vi "top_read_input.vi"(8 "error in (no error)":errorcluster, 10 "Dynamic data":T1, 11 "Input parameters":T2={"Measurement type"=enum."Debug", "Sensor type"=enum."HPK_8in_271ch", "Identifier"="test.txt", "Open after execution?"=FALSE, "Plot after execution?"=FALSE, "Display channel"=0, "Voltage Delay (s)"=0.5, "Switch Delay (s)"=0.01, "VISA resource name source"="", "VISA resource name DMM"="", "VISA resource name LCR"="", "Compliance  Level (A)"=10.0, "Voltage Limit (V)"=1000.0, "Data storage location"="", "Scan voltages"="", "Use source as DMM?"=FALSE, "LCR signal frequenzy (Hz)"=10.0, "DMM device"=enum."Keithley2001", "Sampling number"=1, "Use env. sensors on"=enum."Sensirion sht1x/7x", "Switchboard Handle"=0, "Use Switchboard"=FALSE, "LCR signal voltage (V)"=10000.0, "Repeat"=1, "Scan voltages IV"="", "Scan voltages CV"="", "Hex pad numbers?"=FALSE, "Set measurement type"=enum."Debug", "Custom pad scan"="", "IV voltage Delay (s)"=0.5, "CV voltage Delay (s)"=0.5, "Needle measurement?"=FALSE, "Comments"="test.txt", "LCR signal frequenzy (kHz)"=10.0, "Compliance  Level (uA)"=10.0, "Open Correction Array"=array2304x3[6912 elements], "Current set voltage"=0.0, "Last set voltage"=0.0, "Current channel"=0, "Last OpenCorrection index"=-1, "Total curr/vltg every x steps"=10, "Current channel iteration"=0, "No CV corrections"=FALSE, "Mapfile"="", "Corrfile"="", "IV voltage file"=path "", "CV voltage file"=path "", "IV Switch Delay (s)"=0.01, "CV Switch Delay (s)"=0.01, "Invert polarity"=FALSE, "Set debug dirs"=FALSE, "Is n on p"=FALSE, "Source interlock?"=TRUE, "Voltage file used?"=FALSE, "Pad mask"="", "Mask pad above (uA)"=1.0, "LCR device"=enum."LCR_E4980", "Source device"=enum."Source_2410", "HexPlot binary path"="", "PadReductionFactor"=1.0, "Temperature degC"="", "Fluence [neq]"="", "Annealing [min]"=""} {"CV Switch Delay (s)" format="%#_13g"; "IV Switch Delay (s)" format="%#_13g"; "Last set voltage" format="%#_13g"; "Current set voltage" format="%#_13g"; "CV voltage Delay (s)" format="%#_13g"; "IV voltage Delay (s)" format="%#_13g"; "Voltage Limit (V)" format="%#_13g"; "Voltage Delay (s)" format="%#_13g"; "Switch Delay (s)" format="%#_13g"}) -> (0 "error out":errorcluster, 2 "Dynamic data":T1, 3 "Input parameters":T2={"Measurement type"=enum."Debug", "Sensor type"=enum."HPK_8in_271ch", "Identifier"="test.txt", "Open after execution?"=FALSE, "Plot after execution?"=FALSE, "Display channel"=0, "Voltage Delay (s)"=0.5, "Switch Delay (s)"=0.01, "VISA resource name source"="", "VISA resource name DMM"="", "VISA resource name LCR"="", "Compliance  Level (A)"=10.0, "Voltage Limit (V)"=1000.0, "Data storage location"="", "Scan voltages"="", "Use source as DMM?"=FALSE, "LCR signal frequenzy (Hz)"=10.0, "DMM device"=enum."Keithley2001", "Sampling number"=1, "Use env. sensors on"=enum."Sensirion sht1x/7x", "Switchboard Handle"=0, "Use Switchboard"=FALSE, "LCR signal voltage (V)"=10000.0, "Repeat"=1, "Scan voltages IV"="", "Scan voltages CV"="", "Hex pad numbers?"=FALSE, "Set measurement type"=enum."Debug", "Custom pad scan"="", "IV voltage Delay (s)"=0.5, "CV voltage Delay (s)"=0.5, "Needle measurement?"=FALSE, "Comments"="test.txt", "LCR signal frequenzy (kHz)"=10.0, "Compliance  Level (uA)"=10.0, "Open Correction Array"=array2304x3[6912 elements], "Current set voltage"=0.0, "Last set voltage"=0.0, "Current channel"=0, "Last OpenCorrection index"=-1, "Total curr/vltg every x steps"=10, "Current channel iteration"=0, "No CV corrections"=FALSE, "Mapfile"="", "Corrfile"="", "IV voltage file"=path "", "CV voltage file"=path "", "IV Switch Delay (s)"=0.01, "CV Switch Delay (s)"=0.01, "Invert polarity"=FALSE, "Set debug dirs"=FALSE, "Is n on p"=FALSE, "Source interlock?"=TRUE, "Voltage file used?"=FALSE, "Pad mask"="", "Mask pad above (uA)"=1.0, "LCR device"=enum."LCR_E4980", "Source device"=enum."Source_2410", "HexPlot binary path"="", "PadReductionFactor"=1.0, "Temperature degC"="", "Fluence [neq]"="", "Annealing [min]"=""} {"CV Switch Delay (s)" format="%#_13g"; "IV Switch Delay (s)" format="%#_13g"; "Last set voltage" format="%#_13g"; "Current set voltage" format="%#_13g"; "CV voltage Delay (s)" format="%#_13g"; "IV voltage Delay (s)" format="%#_13g"; "Voltage Limit (V)" format="%#_13g"; "Voltage Delay (s)" format="%#_13g"; "Switch Delay (s)" format="%#_13g"})   [LabVIEW 2020]
doc: "Processes the user input to generate names and constants to be used during program execution."
uses:
  input_params.ctl
  data_dynamic.ctl
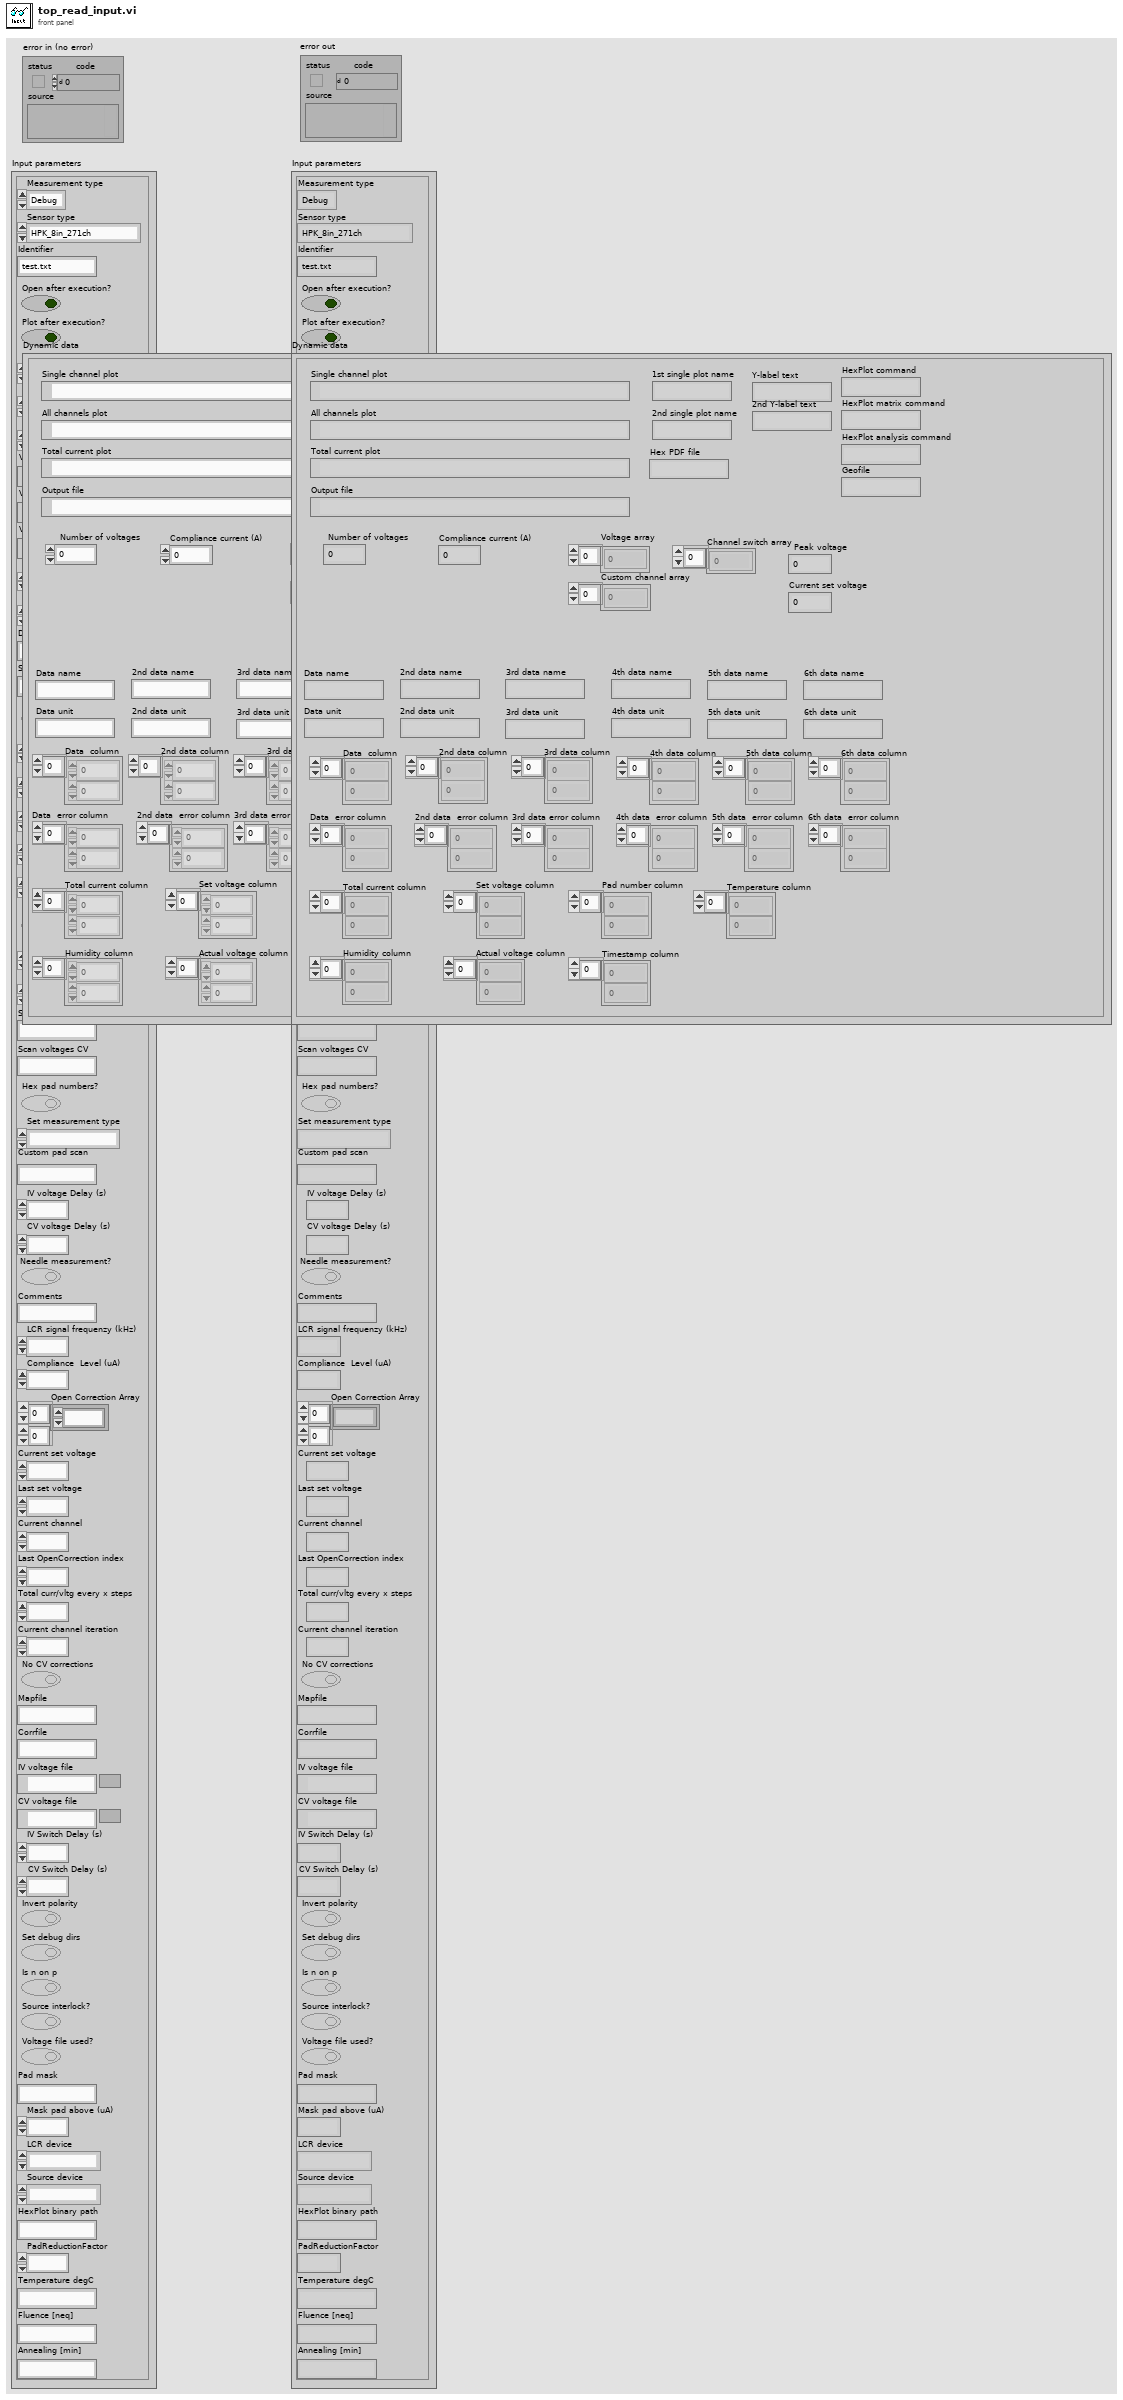
[diagram p1: front panel]
types:
  T1 = typedef "data_dynamic.ctl" = cluster{"Output file":path, "Y-label text":string, "Current set voltage":dbl, "Set voltage column":dbl[], "Pad number column":dbl[], "Data  column":dbl[], "Number of voltages":i32, "Compliance current (A)":dbl, "Geofile":string, "Peak voltage":dbl, "Hex PDF file":string, "Voltage array":dbl[], "Total current column":dbl[], "Timestamp column":dbl[], "Data name":string, "Data unit":string, "2nd data column":dbl[], "2nd data name":string, "2nd data unit":string, "3rd data column":dbl[], "4th data column":dbl[], "3rd data name":string, "3rd data unit":string, "4th data name":string, "4th data unit":string, "Actual voltage column":dbl[], "2nd Y-label text":string, "Single channel plot":path, "Temperature column":dbl[], "Humidity column":dbl[], "Channel switch array":i32[], "1st single plot name":string, "2nd single plot name":string, "All channels plot":path, "HexPlot command":string, "Custom channel array":i32[], "Data  error column":dbl[], "2nd data  error column":dbl[], "3rd data error column":dbl[], "4th data  error column":dbl[], "Total current plot":path, "5th data column":dbl[], "5th data  error column":dbl[], "6th data column":dbl[], "6th data  error column":dbl[], "5th data name":string, "5th data unit":string, "6th data name":string, "6th data unit":string, "HexPlot matrix command":string, "HexPlot analysis command":string}
  T2 = typedef "input_params.ctl" = cluster{"Measurement type":enum16{"IV", "CV", "Debug", "Test_contact"}, "Sensor type":enum16{"HPK_6in_135ch", "HPK_8in_271ch", "IFX_8in_256ch", "Diode", "HPK_6in_239ch", "Full_Matrix", "HPK_8in_271ch_full", "LumiCal", "HPK_8in_444ch", "HPK_8in_198ch_2019", "HPK_8in_MGW_LD_full", "HPK_8in_MGW_LD_a_type_top", "HPK_8in_MGW_LD_a_type_bottom", "HPK_8in_MGW_LD_b_type_left", "HPK_8in_MGW_LD_b_type_right", "HPK_8in_MGW_LD_c_type_left", "HPK_8in_MGW_LD_c_type_right", "HPK_8in_MGW_HD_full", "HPK_8in_MGW_HD_a_type_top", "HPK_8in_MGW_HD_a_type_bottom", "HPK_8in_MGW_HD_b_type_left", "HPK_8in_MGW_HD_b_type_right", "HPK_8in_MGW_HD_c_type_left", "HPK_8in_MGW_HD_c_type_right", "CALICE_6in_256ch"}, "Identifier":string, "Open after execution?":bool, "Plot after execution?":bool, "Display channel":i32, "Voltage Delay (s)":dbl, "Switch Delay (s)":dbl, "VISA resource name source":refnum<visa-resource-name>, "VISA resource name DMM":refnum<visa-resource-name>, "VISA resource name LCR":refnum<visa-resource-name>, "Compliance  Level (A)":dbl, "Voltage Limit (V)":dbl, "Data storage location":string, "Scan voltages":string, "Use source as DMM?":bool, "LCR signal frequenzy (Hz)":dbl, "DMM device":enum16{"Keithley2001", "Keithley2450", "Keithley2410", "Keithley6485", "Keithley6487", "Keithley6517"}, "Sampling number":i32, "Use env. sensors on":enum16{"Sensirion sht1x/7x", "Switch Matrix", "Probecard"}, "Switchboard Handle":u32, "Use Switchboard":bool, "LCR signal voltage (V)":dbl, "Repeat":i32, "Scan voltages IV":string, "Scan voltages CV":string, "Hex pad numbers?":bool, "Set measurement type":enum16{"IV", "CV", "Debug", "Test_contact", "IV+CV"}, "Custom pad scan":string, "IV voltage Delay (s)":dbl, "CV voltage Delay (s)":dbl, "Needle measurement?":bool, "Comments":string, "LCR signal frequenzy (kHz)":dbl, "Compliance  Level (uA)":dbl, "Open Correction Array":dbl[][], "Current set voltage":dbl, "Last set voltage":dbl, "Current channel":i32, "Last OpenCorrection index":i32, "Total curr/vltg every x steps":i32, "Current channel iteration":i32, "No CV corrections":bool, "Mapfile":string, "Corrfile":string, "IV voltage file":path, "CV voltage file":path, "IV Switch Delay (s)":dbl, "CV Switch Delay (s)":dbl, "Invert polarity":bool, "Set debug dirs":bool, "Is n on p":bool, "Source interlock?":bool, "Voltage file used?":bool, "Pad mask":string, "Mask pad above (uA)":dbl, "LCR device":enum16{"LCR_E4980", "AGILENT_4263X"}, "Source device":enum16{"Source_2410", "Source_6487", "Source_2470"}, "HexPlot binary path":string, "PadReductionFactor":dbl, "Temperature degC":string, "Fluence [neq]":string, "Annealing [min]":string}
  T3 = enum16{"HPK_6in_135ch", "HPK_8in_271ch", "IFX_8in_256ch", "Diode", "HPK_6in_239ch", "Full_Matrix", "HPK_8in_271ch_full", "LumiCal", "HPK_8in_444ch", "HPK_8in_198ch_2019", "HPK_8in_MGW_LD_full", "HPK_8in_MGW_LD_a_type_top", "HPK_8in_MGW_LD_a_type_bottom", "HPK_8in_MGW_LD_b_type_left", "HPK_8in_MGW_LD_b_type_right", "HPK_8in_MGW_LD_c_type_left", "HPK_8in_MGW_LD_c_type_right", "HPK_8in_MGW_HD_full", "HPK_8in_MGW_HD_a_type_top", "HPK_8in_MGW_HD_a_type_bottom", "HPK_8in_MGW_HD_b_type_left", "HPK_8in_MGW_HD_b_type_right", "HPK_8in_MGW_HD_c_type_left", "HPK_8in_MGW_HD_c_type_right", "CALICE_6in_256ch"}
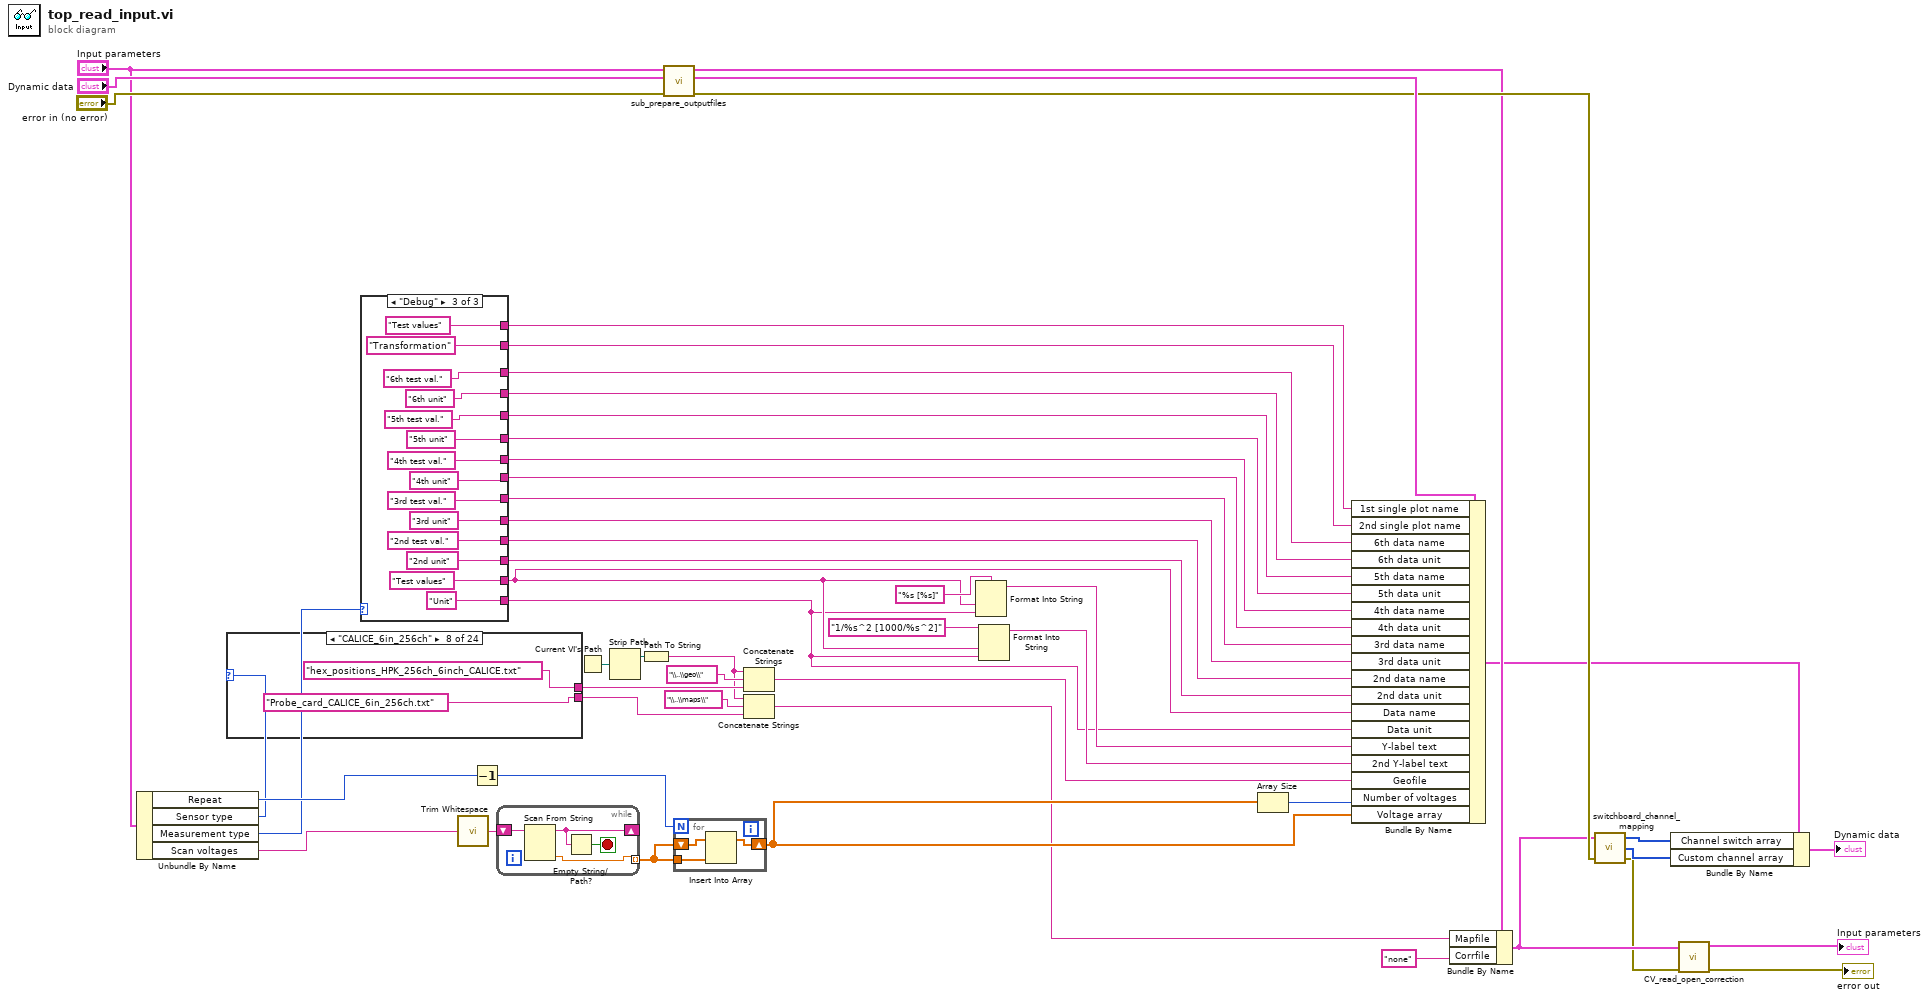
[diagram p0: block diagram]
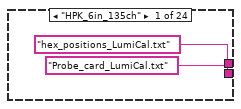
[diagram p2: hidden frame]
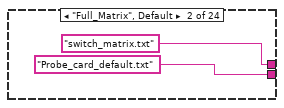
[diagram p3: hidden frame]
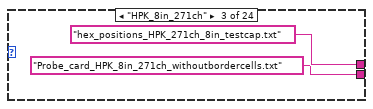
[diagram p4: hidden frame]
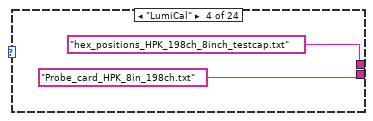
[diagram p5: hidden frame]
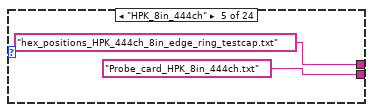
[diagram p6: hidden frame]
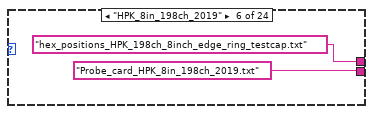
[diagram p7: hidden frame]
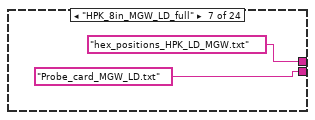
[diagram p8: hidden frame]
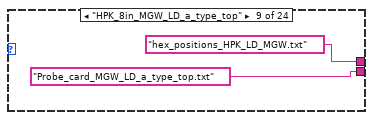
[diagram p9: hidden frame]
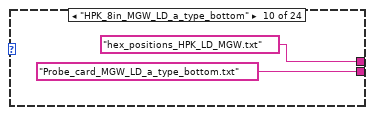
[diagram p10: hidden frame]
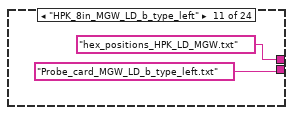
[diagram p11: hidden frame]
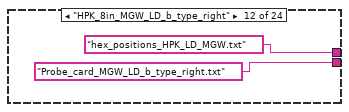
[diagram p12: hidden frame]
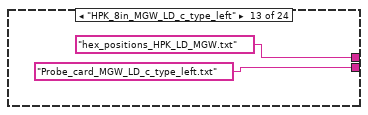
[diagram p13: hidden frame]
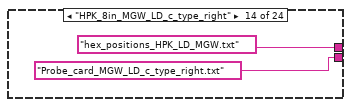
[diagram p14: hidden frame]
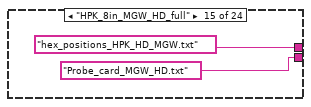
[diagram p15: hidden frame]
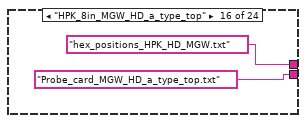
[diagram p16: hidden frame]
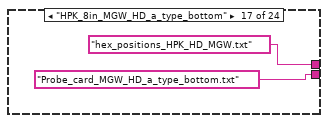
[diagram p17: hidden frame]
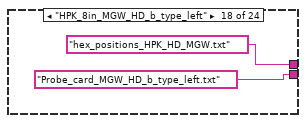
[diagram p18: hidden frame]
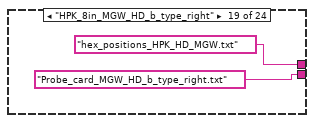
[diagram p19: hidden frame]
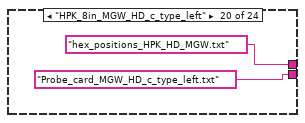
[diagram p20: hidden frame]
diagram:
  n1 = Unbundle By Name("Input parameters") -> ("Repeat"=w36:i32, "Sensor type"=w16:T3, "Measurement type"=w27:enum16{"IV", "CV", "Debug", "Test_contact"}, "Scan voltages"=w31:string)
  n2 = case shown="\"CALICE_6in_256ch\"" w16 {
    tunnel: ["hex_positions_LumiCal.txt" ("name or relative path") "switch_matrix.txt" ("name or relative path") "hex_positions_HPK_271ch_8in_testcap.txt" ("name or relative path") "hex_positions_HPK_198ch_8inch_testcap.txt" ("name or relative path") "hex_positions_HPK_444ch_8in_edge_ring_testcap.txt" ("name or relative path") "hex_positions_HPK_198ch_8inch_edge_ring_testcap.txt" ("name or relative path") "hex_positions_HPK_LD_MGW.txt" ("name or relative path") "hex_positions_HPK_256ch_6inch_CALICE.txt" ("name or relative path") "hex_positions_HPK_LD_MGW.txt" ("name or relative path") "hex_positions_HPK_LD_MGW.txt" ("name or relative path") "hex_positions_HPK_LD_MGW.txt" ("name or relative path") "hex_positions_HPK_LD_MGW.txt" ("name or relative path") "hex_positions_HPK_LD_MGW.txt" ("name or relative path") "hex_positions_HPK_LD_MGW.txt" ("name or relative path") "hex_positions_HPK_HD_MGW.txt" ("name or relative path") "hex_positions_HPK_HD_MGW.txt" ("name or relative path") "hex_positions_HPK_HD_MGW.txt" ("name or relative path") "hex_positions_HPK_HD_MGW.txt" ("name or relative path") "hex_positions_HPK_HD_MGW.txt" ("name or relative path") "hex_positions_HPK_HD_MGW.txt" ("name or relative path") "hex_positions_HPK_HD_MGW.txt" ("name or relative path") "hex_positions_HPK_271ch_8in_testcap.txt" ("name or relative path") "hex_positions_HPK_239ch_6in_testcap.txt" ("name or relative path") "hex_positions_IFX_256ch_8in.txt" ("name or relative path")] -> w51
    tunnel: ["Probe_card_LumiCal.txt" ("name or relative path") "Probe_card_default.txt" ("name or relative path") "Probe_card_HPK_8in_271ch_withoutbordercells.txt" ("name or relative path") "Probe_card_HPK_8in_198ch.txt" ("name or relative path") "Probe_card_HPK_8in_444ch.txt" ("name or relative path") "Probe_card_HPK_8in_198ch_2019.txt" ("name or relative path") "Probe_card_MGW_LD.txt" ("name or relative path") "Probe_card_CALICE_6in_256ch.txt" ("name or relative path") "Probe_card_MGW_LD_a_type_top.txt" ("name or relative path") "Probe_card_MGW_LD_a_type_bottom.txt" ("name or relative path") "Probe_card_MGW_LD_b_type_left.txt" ("name or relative path") "Probe_card_MGW_LD_b_type_right.txt" ("name or relative path") "Probe_card_MGW_LD_c_type_left.txt" ("name or relative path") "Probe_card_MGW_LD_c_type_right.txt" ("name or relative path") "Probe_card_MGW_HD.txt" ("name or relative path") "Probe_card_MGW_HD_a_type_top.txt" ("name or relative path") "Probe_card_MGW_HD_a_type_bottom.txt" ("name or relative path") "Probe_card_MGW_HD_b_type_left.txt" ("name or relative path") "Probe_card_MGW_HD_b_type_right.txt" ("name or relative path") "Probe_card_MGW_HD_c_type_left.txt" ("name or relative path") "Probe_card_MGW_HD_c_type_right.txt" ("name or relative path") "Probe_card_HPK_8in_271ch.txt" ("name or relative path") "Probe_card_HPK_6in_239ch.txt" ("name or relative path") "Probe_card_IFX_8in.txt" ("name or relative path")] -> w14
    frame "HPK_6in_135ch" {
    }
    frame "Full_Matrix", Default {
    }
    frame "HPK_8in_271ch" {
    }
    frame "LumiCal" {
    }
    frame "HPK_8in_444ch" {
    }
    frame "HPK_8in_198ch_2019" {
    }
    frame "HPK_8in_MGW_LD_full" {
    }
    frame "CALICE_6in_256ch" {
    }
    frame "HPK_8in_MGW_LD_a_type_top" {
    }
    frame "HPK_8in_MGW_LD_a_type_bottom" {
    }
    frame "HPK_8in_MGW_LD_b_type_left" {
    }
    frame "HPK_8in_MGW_LD_b_type_right" {
    }
    frame "HPK_8in_MGW_LD_c_type_left" {
    }
    frame "HPK_8in_MGW_LD_c_type_right" {
    }
    frame "HPK_8in_MGW_HD_full" {
    }
    frame "HPK_8in_MGW_HD_a_type_top" {
    }
    frame "HPK_8in_MGW_HD_a_type_bottom" {
    }
    frame "HPK_8in_MGW_HD_b_type_left" {
    }
    frame "HPK_8in_MGW_HD_b_type_right" {
    }
    frame "HPK_8in_MGW_HD_c_type_left" {
    }
    frame "HPK_8in_MGW_HD_c_type_right" {
    }
    frame "HPK_8in_271ch_full" {
    }
    frame "HPK_6in_239ch" {
    }
    frame "IFX_8in_256ch" {
    }
  }
  n3 = case shown="\"Debug\"" w27 {
    tunnel: ["Current" "Cs" "Test values"] -> w39
    tunnel: ["nA" "pF" "Unit"] -> w26
    tunnel: [w100 "Cp" "2nd test val."] -> w22
    tunnel: [w100 "pF" "2nd unit"] -> w45
    tunnel: [w100 "Ohm" "3rd unit"] -> w44
    tunnel: [w100 "Impedance" "3rd test val."] -> w43
    tunnel: [w100 "Rad" "4th unit"] -> w42
    tunnel: [w100 "Phase" "4th test val."] -> w41
    tunnel: ["Current" "Capacitance" "Test values"] -> w32
    tunnel: ["n/a" "Transformation" "Transformation"] -> w33
    tunnel: [w100 "pF" "5th unit"] -> w20
    tunnel: [w100 "Cs uncorr." "5th test val."] -> w19
    tunnel: [w100 "pF" "6th unit"] -> w18
    tunnel: [w100 "Cp uncorr." "6th test val."] -> w17
    frame "IV", Default {
      w100 = "n/a"
    }
    frame "CV" {
    }
    frame "Debug" {
    }
  }
  n4 = call <vilib>:"Trim Whitespace.vi"("string"=w31) -> ("trimmed string"=w49:string)  [unwired: 1 in]
  n5 = Decrement(x=w36) -> (x-1=w34:i32)
  n6 = while {
    shift-right: [w135] -> _
    shift-left: w49 -> [w136]
    tunnel: [w133] -> w35 mode=indexing
    stop <- w134 stop-if-true
    n7 = Scan From String(input string=w136) -> (remaining string=w135:string, output 1=w133:dbl)  [unwired: 4 in, 2 out]
    n8 = Empty String/Path?(string/path=w135) -> (empty?=w134:bool)
  }
  n9 = Current VI's Path() -> (path=w48:path)
  n10 = Strip Path(path=w48) -> (stripped path=w47:path)  [unwired: 1 out]
  n11 = Path To String(path=w47) -> (string=w7:string)
  n12 = call "sub_prepare_outputfiles.vi"("error in"="error in (no error)", "Dynamic data in"="Dynamic data", "Input parameters"="Input parameters") -> ("error out"=w24:errorcluster, "Dynamic data out"=w28:T1, "Input parameters out"=w23:T2)  [unwired: 6 in]
  n13 = for {
    N: w34 -> [_]
    tunnel: w35 -> [w138]
    shift-right: [w137] -> w21
    shift-left: w35 -> [w139]
    n14 = Insert Into Array(array=w139, new element=w138) -> (w137:dbl[])  [unwired: 1 in]
  }
  n15 = Concatenate Strings(w7, "\\..\\geo\\" ("string"), w51) -> (w25:string)
  n16 = Concatenate Strings(w7, "\\..\\maps\\" ("string"), w14) -> (w12:string)
  n17 = Format Into String(format string="%s [%s]", w39, w26) -> (resulting string=w37:string)  [unwired: 2 in, 1 out]
  n18 = Format Into String(format string="1/%s^2 [1000/%s^2]", w39, w26) -> (resulting string=w38:string)  [unwired: 2 in, 1 out]
  n19 = Array Size(array=w21) -> (size(s)=w50:i32)
  n20 = Bundle By Name(cluster=w28, "1st single plot name"=w32, "2nd single plot name"=w33, "6th data name"=w17, "6th data unit"=w18, "5th data name"=w19, "5th data unit"=w20, "4th data name"=w41, "4th data unit"=w42, "3rd data name"=w43, "3rd data unit"=w44, "2nd data name"=w22, "2nd data unit"=w45, "Data name"=w39, "Data unit"=w26, "Y-label text"=w37, "2nd Y-label text"=w38, "Geofile"=w25, "Number of voltages"=w50, "Voltage array"=w21) -> (w10:T1)
  n21 = Bundle By Name(cluster=w23, "Mapfile"=w12, "Corrfile"="none" ("name or relative path")) -> (w6:T2)
  n22 = call "switchboard_channel_mapping.vi"("error in"=w24, "Input parameters"=w6) -> ("error out"=w4:errorcluster, "Custom pad array"=w8:i32[], "Channel switch array"=w11:i32[])  [unwired: 1 in]
  n23 = Bundle By Name(cluster=w10, "Channel switch array"=w11, "Custom channel array"=w8) -> (→"Dynamic data":T1)
  n24 = call "CV_read_open_correction.vi"("error in"=w4, "Input parameters in"=w6) -> ("error out"=→"error out":errorcluster, "Input parameters out"=→"Input parameters":T2)  [unwired: 8 in]
